vi "Lift Eject.vi"() -> ()   [LabVIEW 2014]
uses:
  Begin/Global RefNums.vi
  Begin/Global Variables.vi
panel:
  in  "Range":dbl=0.2 format="%#_13g"
  out "Voltage":dbl
  in  "Silver":dbl
  in  "Yellow":dbl
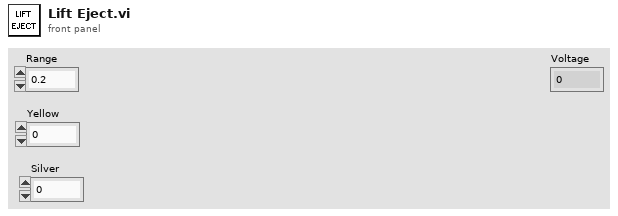
[diagram p1: front panel]
types:
  T1 = typedef "WPI_AnalogChannelDevRef.ctl" = cluster{"DevStatus":errorcluster, "Controller":T2, "Analog Channel":T3}
  T2 = typedef "FPGA_TypedefAnalogModule.ctl" = enum16{"Controller 1"}
  T3 = typedef "FPGA_AIChannel.ctl" = enum8{"AI 0", "AI 1", "AI 2", "AI 3", "AI MXP 0", "AI MXP 1", "AI MXP 2", "AI MXP 3", "Invalid"}
  T4 = typedef "WPI_MotorControlDeviceRef.ctl" = cluster{"DeviceStatus":errorcluster, "Type":T5, "PWM":cluster{"Controller":T6, "PWM Channel":T7, "DeadBand":T8}, "CAN":cluster{"Device Number":u8, "Control Mode":T9, "Semaphore":T10, "Max Vout":dbl, "TalonSRX Control Mode":T11}, "Invert":bool, "TransformRef":T12, "InvTransformRef":T12}
  T5 = typedef "WPI_MotorControlType.ctl" = enum16{"PWM", "CAN", "CANTalonSRX"}
  T6 = typedef "FPGA_TypedefDigitalModule.ctl" = enum16{"Controller 1"}
  T7 = typedef "FPGA_DIOPWMChannel.ctl" = enum8{"PWM 0", "PWM 1", "PWM 2", "PWM 3", "PWM 4", "PWM 5", "PWM 6", "PWM 7", "PWM 8", "PWM 9", "PWM MXP 0", "PWM MXP 1", "PWM MXP 2", "PWM MXP 3", "PWM MXP 4", "PWM MXP 5", "PWM MXP 6", "PWM MXP 7", "PWM MXP 8", "PWM MXP 9", "Invalid"}
  T8 = typedef "WPI_PWMDeadband.ctl" = cluster{"Name":string, "maxPositivePwm":i32, "minPositivePwm":i32, "centerPwm":i32, "maxNegativePwm":i32, "minNegativePwm":i32, "angularRange":u16}
  T9 = typedef "WPI_CANJaguar_ControlMode.ctl" = enum8{"Percent VBus", "Current", "Speed", "Position", "Voltage"}
  T10 = typedef "Semaphore RefNum" = refnum<k1>
  T11 = typedef "WPI_CANTalonSRX_APIControlMode.ctl" = enum8{"Percent VBus", "Speed", "Position", "Slave", "Unchanged / Invalid"}
  T12 = typedef "WPI_PWMTransform_ConPane.ctl" = refnum<vi>
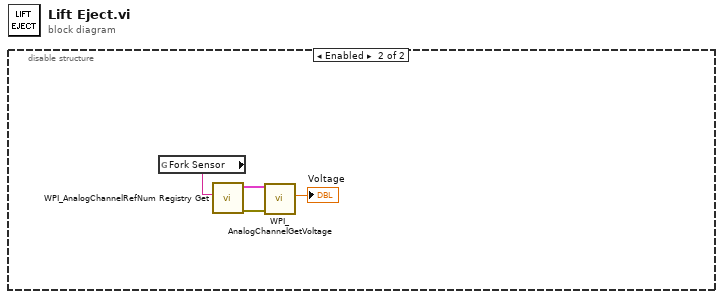
[diagram p0: block diagram]
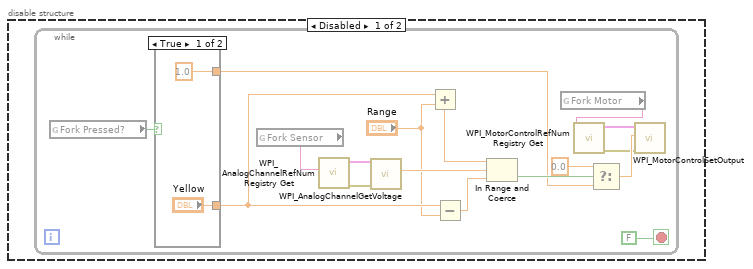
[diagram p2: hidden frame]
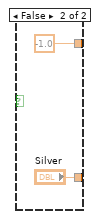
[diagram p3: hidden frame]
diagram:
  n1 = disable-structure shown="Enabled" {
    frame Disabled {
      n2 = while {
        stop <- FALSE stop-if-true
        n3 = global read "Global Variables.vi" "Fork Pressed?"() -> (w3:bool)
        n4 = case shown="True" w3 {
          tunnel: [1.0 ("t") -1.0 ("t")] -> w1
          tunnel: ["Yellow" "Silver"] -> w6
          frame True {
          }
          frame False {
          }
        }
        n5 = global read "Global RefNums.vi" "Fork Sensor"() -> (w10:string)
        n6 = call <vilib>:"WPI_AnalogChannelRefNum Registry Get.vi"("refnum name"=w10) -> ("error out"=w9:errorcluster, "AIDeviceRef"=w8:T1)  [unwired: 9 in]
        n7 = call <vilib>:"WPI_AnalogChannelGetVoltage.vi"("error in (no error)"=w9, "AIDeviceRef"=w8) -> ("Voltage"=w17:dbl)  [unwired: 7 in, 2 out]
        n8 = Add(x=w6, y="Range") -> (x+y=w15:dbl)
        n9 = Subtract(x=w6, y="Range") -> (x-y=w16:dbl)
        n10 = In Range and Coerce(upper limit=w15, x=w17, lower limit=w16) -> (In Range?=w7:bool)  [unwired: 1 out]
        n11 = global read "Global RefNums.vi" "Fork Motor"() -> (w13:string)
        n12 = call <vilib>:"WPI_MotorControlRefNum Registry Get.vi"("refnum name"=w13) -> ("error out"=w12:errorcluster, "MotorControlDevRef"=w11:T4)  [unwired: 9 in]
        n13 = Select(t=0.0 ("f"), s=w7, f=w1) -> (s? t:f=w14:dbl)
        n14 = call <vilib>:"WPI_MotorControlSetOutput.vi"("error in (no error)"=w12, "Output"=w14, "MotorControlDevRef"=w11) -> ()  [unwired: 6 in, 3 out]
      }
    }
    frame Enabled {
      n15 = global read "Global RefNums.vi" "Fork Sensor"() -> (w23:string)
      n16 = call <vilib>:"WPI_AnalogChannelRefNum Registry Get.vi"("refnum name"=w23) -> ("error out"=w24:errorcluster, "AIDeviceRef"=w25:T1)  [unwired: 9 in]
      n17 = call <vilib>:"WPI_AnalogChannelGetVoltage.vi"("error in (no error)"=w24, "AIDeviceRef"=w25) -> ("Voltage"=→"Voltage":dbl)  [unwired: 7 in, 2 out]
    }
  }
